vi "HS-Tester - Transmit QAM Data.vi"(8 "error in (no error)":errorcluster, 9 "Simulation Data":T1={"PowerOn"=TRUE, "Battery"=TRUE, "Antenna"=TRUE, "Microphone"=TRUE, "Speakers"=TRUE, "Buttons"=TRUE, "LCD"=enum."Passing Image"}, 10 "QAM Data In":cluster{dbl[], dbl[]}, 11 "VISA resource name":refnum<visa-resource-name>) -> (0 "error out":errorcluster, 3 "VISA resource name out":refnum<visa-resource-name>)   [LabVIEW 2019]
uses:
  Public/Documents/National Instruments/TestStand 2019 (64-bit)/Examples/Demos/Mobile Device Test/LabVIEW/Source/Support/Simulation Data.ctl
  Public/Documents/National Instruments/TestStand 2019 (64-bit)/Examples/Demos/Mobile Device Test/LabVIEW/Source/Support/Antenna Simulation States.ctl
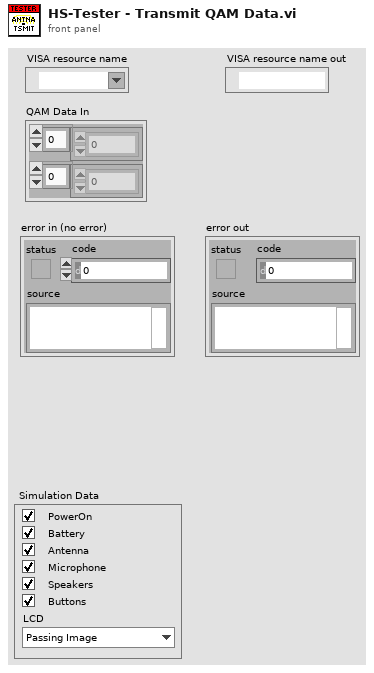
[diagram p1: front panel]
types:
  T1 = typedef "Simulation Data.ctl" = cluster{"PowerOn":bool, "Battery":bool, "Antenna":bool, "Microphone":bool, "Speakers":bool, "Buttons":bool, "LCD":enum16{"Passing Image", "Dead Pixels", "Incorrect Brightness"}}
  T2 = typedef "Antenna Simulation States.ctl" = enum16{"Simulate Transmit Antenna QAM Data", "Simulate Receive Antenna QAM Data"}
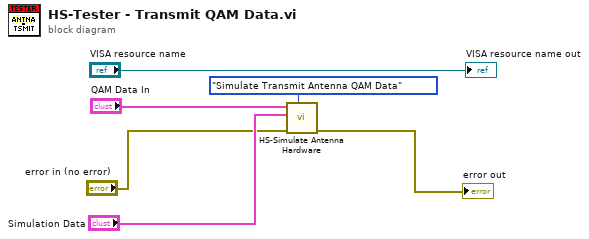
[diagram p0: block diagram]
diagram:
  n1 = call "HS-Simulate Antenna Hardware.vi"("Command to Simulate"=Antenna_Simulation_States."Simulate Transmit Antenna QAM Data", "error in (no error)"="error in (no error)", "Simulation Data"="Simulation Data", "QAM Data In"="QAM Data In") -> ("error out"=→"error out":errorcluster)  [unwired: 6 in, 1 out]
  "VISA resource name out" <- "VISA resource name"
